vi "Error - Reversed I2C.vi"   [LabVIEW 2020, in "CTI-Scratchpad.lvlib"]
uses:
  CTI-Scratchpad.lvlib
  CTI/I2C Number.ctl
  CTI/GPIO Number.ctl
  CTI/Session/Session.lvclass
  CTI/VisaComms/VisaComms.lvclass
  CTI/CTI.lvlib
panel:
  # "Configure/run this on BD."
types:
  T1 = typedef "CTI.lvlib/GPIO Number.ctl" = i8
  T2 = typedef "CTI.lvlib/I2C Number.ctl" = i8
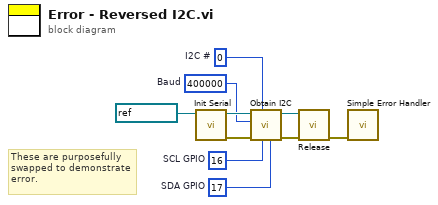
[diagram p0: block diagram]
diagram:
  w4 = T1 17  # SDA GPIO
  w5 = T1 16  # SCL GPIO
  w6 = T2 0  # I2C #
  w7 = u32 400000  # Baud
  # "These are purposefully swapped to demonstrate error."
  n1 = call "Init Serial.vi"("VISA resource name in"=refnum<visa-resource-name> "COM5" ("Port")) -> ("error out"=w8:errorcluster, "Session"=w9:refnum<class "Session.lvclass">)  [unwired: 8 in, 1 out]
  n2 = call "Obtain I2C.vi"("SDA GPIO"=w4, "SCL GPIO"=w5, "I2C #"=w6, "error in (no error)"=w8, "Baud"=w7, "Session in"=w9) -> ("error out"=w3:errorcluster, "Session out"=w2:refnum<class "Session.lvclass">)  [unwired: 4 in]
  n3 = call-dynamic "Release.vi"("error in (no error)"=w3, "Session in"=w2) -> ("error out"=w1:errorcluster)  [unwired: 9 in]
  n4 = call <vilib>:"Simple Error Handler.vi"("error in (no error)"=w1) -> ()  [unwired: 4 in, 5 out]
